vi "00 Main (three phase) (2017).vi"() -> ()   [LabVIEW 2017]
uses:
  <vilib>/DAQmx/read.llb/DAQmx Read (Analog 1D Wfm NChan NSamp).vi
  <vilib>/DAQmx/miscellaneous.llb/DAQmx Fill In Error Info.vi
panel:
  out "Error out (DAQ Loop)":errorcluster
  out "DAQ Loop Iterations":i32
  out "Raw DAQ Output":dynamicdata(graph)=[{"t0"=timestamp(3367839419.335167 s since 1904-01-01), "dt"=0.00016666666666666663, "Y"=array[240 elements], "attributes"=variant("NI_ChannelName"=variant(string "Voltage_0"), "NI_UnitDescription"=variant(string "Volts"))}, {"t0"=timestamp(3367839419.3351874 s since 1904-01-01), "dt"=0.00016666666666666663, "Y"=array[240 elements], "attributes"=variant("NI_ChannelName"=variant(string "Voltage_1"), "NI_UnitDescription"=variant(string "Volts"))}, {"t0"=timestamp(3367839419.3352084 s since 1904-01-01), "dt"=0.00016666666666666663, "Y"=array[240 elements], "attributes"=variant("NI_ChannelName"=variant(string "Voltage_2"), "NI_UnitDescription"=variant(string "Volts"))}]
  in  "All Stop!":bool
  out "Frequency 2":dynamicdata(graph)=[{"t0"=timestamp(3424329819.6880417 s since 1904-01-01), "dt"=0.00016666666666666663, "Y"=[50.00644377121546], "attributes"=variant("NI_ChannelName"=variant(string "Detected Frequency"))}, {"t0"=timestamp(3424329819.6880627 s since 1904-01-01), "dt"=0.00016666666666666663, "Y"=[49.993846178541475], "attributes"=variant("NI_ChannelName"=variant(string "Detected Frequency"))}, {"t0"=timestamp(3424329819.6880836 s since 1904-01-01), "dt"=0.00016666666666666663, "Y"=[49.994041382621866], "attributes"=variant("NI_ChannelName"=variant(string "Detected Frequency"))}] caption="Frequency"
  out "Phase 2":dynamicdata(graph)=[{"t0"=timestamp(3424329819.6880417 s since 1904-01-01), "dt"=0.00016666666666666663, "Y"=[-19.090260250465658], "attributes"=variant("NI_ChannelName"=variant(string "Detected Phase"))}, {"t0"=timestamp(3424329819.6880627 s since 1904-01-01), "dt"=0.00016666666666666663, "Y"=[-138.45601955575555], "attributes"=variant("NI_ChannelName"=variant(string "Detected Phase"))}, {"t0"=timestamp(3424329819.6880836 s since 1904-01-01), "dt"=0.00016666666666666663, "Y"=[102.37498697247455], "attributes"=variant("NI_ChannelName"=variant(string "Detected Phase"))}] caption="Frequency"
  out "Frequency":dbl format="%.2f"
  out "Amplitude":dbl format="%.2f"
  out "Phase":dbl format="%.2f"
  out "Acquisition Time":timestamp
  out "Voltage Waveform":dynamicdata(graph)=[{"t0"=timestamp(3424329819.638042 s since 1904-01-01), "dt"=0.00016666666666666663, "Y"=array[300 elements]}, {"t0"=timestamp(3424329819.6380625 s since 1904-01-01), "dt"=0.00016666666666666663, "Y"=array[300 elements]}, {"t0"=timestamp(3424329819.6380835 s since 1904-01-01), "dt"=0.00016666666666666663, "Y"=array[300 elements]}]
  out "IP":string
  out "Port":i32
  out "Transmitted Data":string
  out "Stop":bool
  out "Elements in Acquisition Buffer":i32
  # "V1.2 - PFI0 (Three Phase)"
  # "50.5"
  # "49.5"
  # "The code and design of this VI are licensed \nunder the terms of the New BSD License.\nPlease see the VI documentation or License.txt\nfor more details.\n\nCopyright (c) 2012, David Laverty\nwww.OpenPMU.org"
  # "180"
  # "-180"
  # "Configuration Information:\n\nThe ID and IP address to which the OpenPMU sends data is configured by 'C:\\PMUconfig.ini'.  If this doesn't exist, create it.\n\nCopy and paste the blue text below without the dashed lines into PMUconfig.ini.\n\n[Telecoms]\nID=PMU123\nIP=192.168.1.100\nPort=40001\n\nIP and Port may be any values within normal IPv4 range.  ID should be six alpha-numeric characters."
  # "Debug Stuff ( you're not supposed to find this :P )"
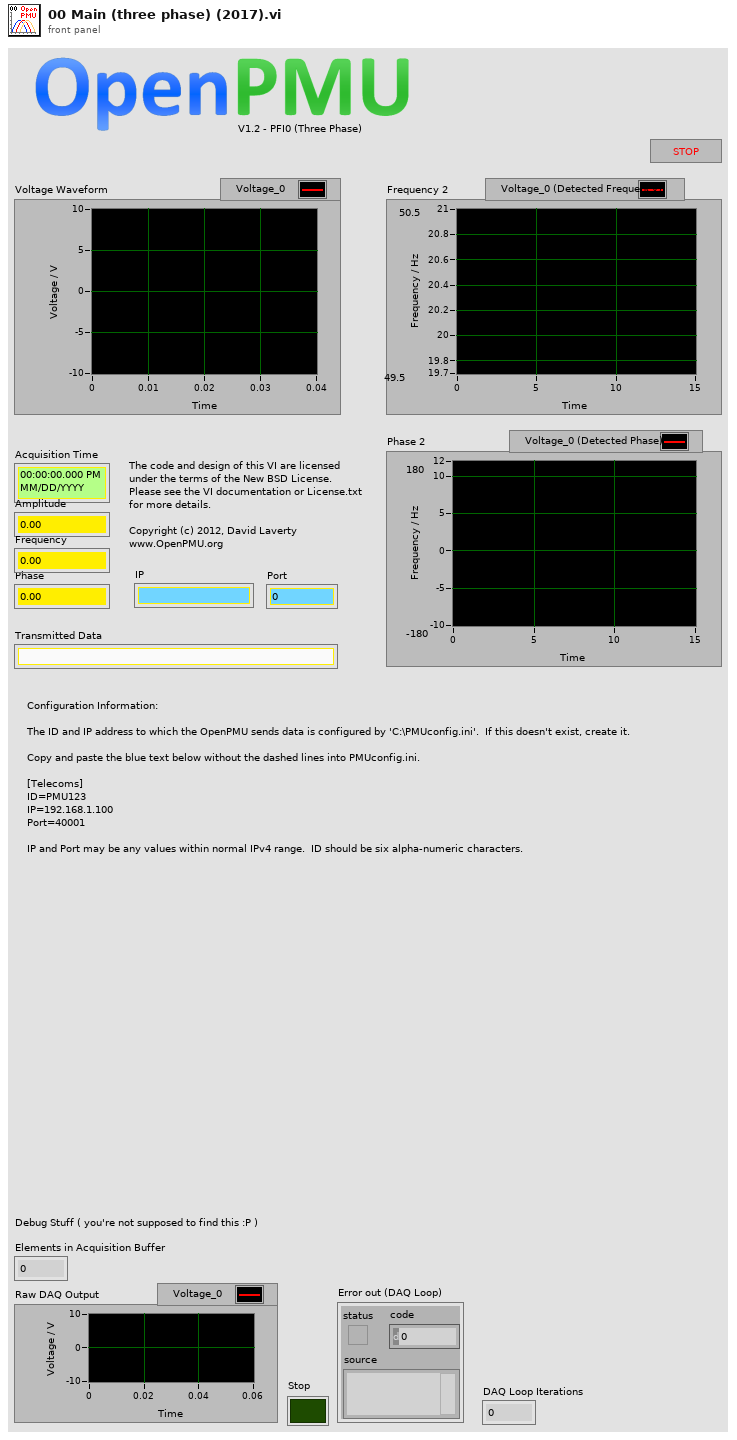
[diagram p1: front panel]
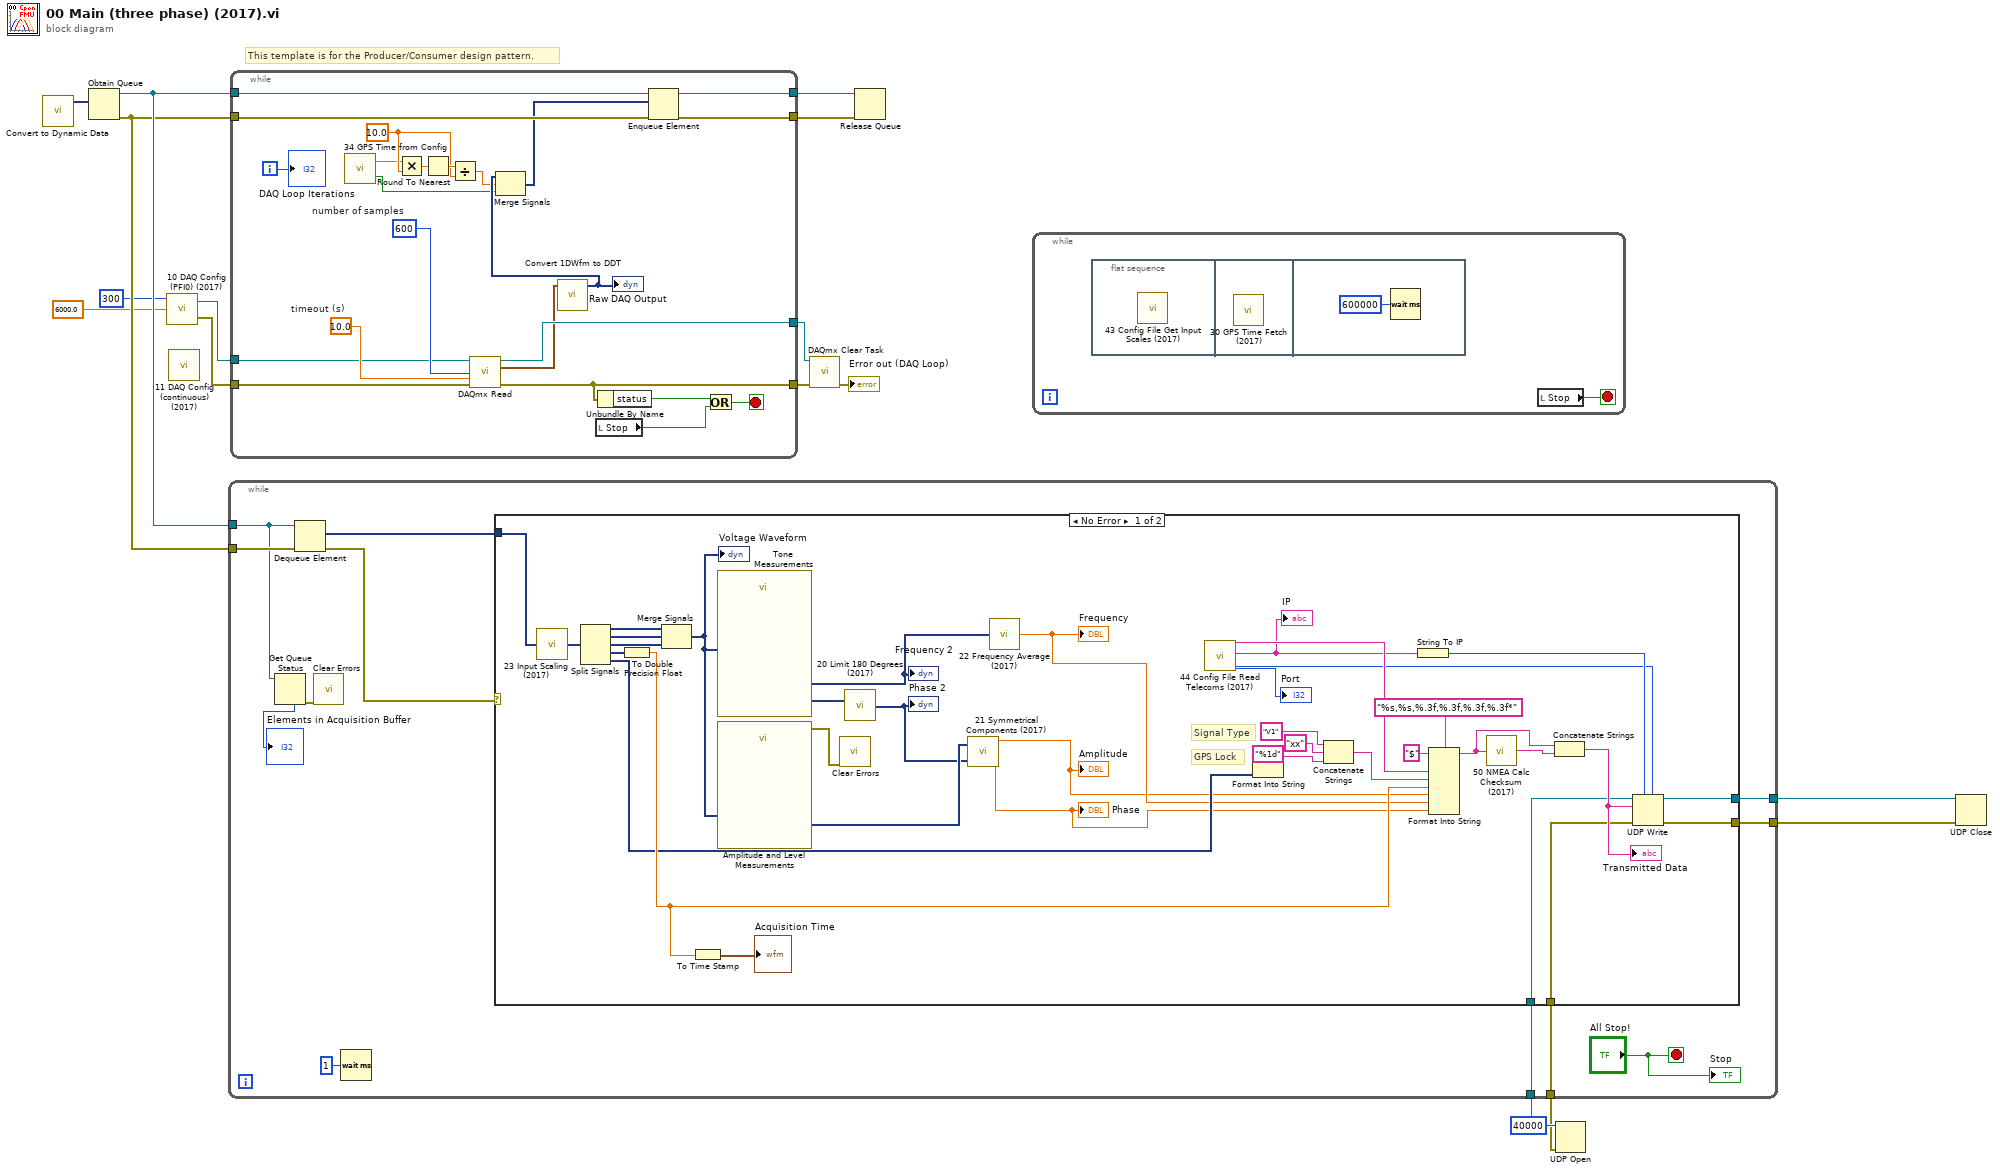
[diagram p0: block diagram]
diagram:
  # "This template is for the Producer/Consumer design pattern."
  n1 = call "Convert to Dynamic Data"() -> ("Dynamic Data Type"=w14:dynamicdata)  [unwired: 4 in]
  n2 = Obtain Queue(element data type=w14) -> (queue out=w11:refnum<queue>, error out=w10:errorcluster)  [unwired: 4 in, 1 out]
  n3 = call "10 DAQ Config (PFI0) (2017).vi"("rate"=6000.0, "number of samples"=300) -> ("Error Out"=w1:errorcluster, "task out"=w2:refnum<k21>)  [unwired: 1 in]
  n4 = call "11 DAQ Config (continuous) (2017).vi"() -> ()  [unwired: 1 in, 2 out]
  n5 = while {
    tunnel: w1 -> [w26]
    tunnel: w2 -> [w27]
    tunnel: [w37] -> w17
    tunnel: [w36] -> w16
    tunnel: w11 -> [w31]
    tunnel: w10 -> [w30]
    tunnel: [w29] -> w13
    tunnel: [w28] -> w12
    i -> [w35]
    stop <- w34 stop-if-true
    w20 = 10.0 ("y")
    w38 = 10.0  # timeout (s)
    w40 = 600  # number of samples
    n6 = call "34 GPS Time from Config.vi"() -> ("GPS Lock"=w18:bool, "Time"=w19:dbl)  [unwired: 2 in]
    n7 = Multiply(x=w19, y=w20) -> (x*y=w23:dbl)
    n8 = Round To Nearest(number=w23) -> (nearest integer value=w22:dbl)
    n9 = Divide(x=w22, y=w20) -> (x/y=w21:dbl)
    n10 = call-poly <vilib>:"DAQmx Read.vi"("task/channels in"=w27, "number of samples per channel"=w40, "timeout"=w38, "error in"=w26) -> ("task out"=w37:refnum<k21>, "data"=w33:waveform(dbl)[], "error out"=w36:errorcluster)  [unwired: 9 in]
    n11 = call <vilib>:"Convert 1DWfm to DDT.vi"("Array of Waveforms"=w33) -> ("Dynamic Data Type"=w25:dynamicdata)  [unwired: 3 in]
    "Raw DAQ Output" <- w25
    n12 = Merge Signals(w25, w21, w18) -> (w24:dynamicdata)
    n13 = local read "Stop"() -> (w32:bool)
    n14 = Unbundle By Name(w36) -> ("status"=w39:bool)
    n15 = Enqueue Element(queue=w31, element=w24, error in (no error)=w30) -> (queue out=w29:refnum<queue>, error out=w28:errorcluster)  [unwired: 1 in, 1 out]
    n16 = Or(x=w39, y=w32) -> (x .or. y?=w34:bool)
    "DAQ Loop Iterations" <- w35
  }
  n17 = call <vilib>:"DAQmx Clear Task.vi"("task in"=w17, "error in"=w16) -> ("error out"=→"Error out (DAQ Loop)":errorcluster)  [unwired: 13 in]
  n18 = Release Queue(queue=w13, error in (no error)=w12) -> ()  [unwired: 1 in, 3 out]
  n19 = while {
    stop <- w41 stop-if-true
    n20 = flat-sequence {
      frame #0 {
        n21 = call "43 Config File Get Input Scales (2017).vi"() -> ()  [unwired: 1 in]
      }
      frame #1 {
        n22 = call "30 GPS Time Fetch (2017).vi"() -> ()  [unwired: 1 in]
      }
      frame #2 {
        n23 = Wait (ms)(milliseconds to wait=u32 600000) -> ()  [unwired: 1 out]
      }
    }
    n24 = local read "Stop"() -> (w41:bool)
  }
  n25 = UDP Open(11:u16 40000 ("port")) -> (port=w8:refnum<k16>, 0:w7:errorcluster)  [unwired: 4 in, 1 out]
  n26 = while {
    tunnel: w11 -> [w48]
    tunnel: w10 -> [w50]
    tunnel: w8 -> [w47]
    tunnel: w7 -> [w46]
    tunnel: [w45] -> w6
    tunnel: [w44] -> w5
    stop <- "All Stop!" stop-if-true
    n27 = Get Queue Status(queue=w48) -> (error out=w43:errorcluster, # elements in queue=→"Elements in Acquisition Buffer":i32)  [unwired: 2 in, 6 out]
    n28 = Dequeue Element(queue=w48, error in (no error)=w50) -> (element=w51:dynamicdata, error out=w52:errorcluster)  [unwired: 1 in, 2 out]
    n29 = call <vilib>:"Clear Errors.vi"("error in (no error)"=w43) -> ()  [unwired: 5 in, 2 out]
    n30 = Wait (ms)(milliseconds to wait=u32 1) -> ()  [unwired: 1 out]
    n31 = case shown="No Error" w52 {
      tunnel: w51 -> [w56 _]
      tunnel: w47 -> [w84 w92]
      tunnel: w46 -> [w83 w91]
      tunnel: [w82 w92] -> w45
      tunnel: [w81 w91] -> w44
      frame No Error {
        # "GPS Lock"
        # "Signal Type"
        n32 = call "23 Input Scaling (2017).vi"("Input (Raw)"=w56) -> ("Output (Scaled)"=w55:dynamicdata)
        n33 = Split Signals(w55) -> (w69:dynamicdata, w70:dynamicdata, w71:dynamicdata, w80:dynamicdata, w78:dynamicdata)  [unwired: 5 in]
        n34 = To Double Precision Float(number=w80) -> (double precision float=w79:dbl)
        n35 = Merge Signals(w69, w70, w71) -> (w72:dynamicdata)
        "Voltage Waveform" <- w72
        n36 = To Time Stamp(1:w79) -> (0:→"Acquisition Time":timestamp)
        n37 = call "Tone Measurements"("Signals"=w72) -> ("Phase"=w68:dynamicdata, "Frequency"=w67:dynamicdata)  [unwired: 7 in, 2 out]
        "Frequency 2" <- w67
        n38 = call "Amplitude and Level Measurements"("Signals"=w72) -> ("Cycle RMS"=w65:dynamicdata, "error out"=w90:errorcluster)  [unwired: 13 in]
        n39 = call <vilib>:"Clear Errors.vi"("error in (no error)"=w90) -> ()  [unwired: 5 in, 2 out]
        n40 = call "20 Limit 180 Degrees (2017).vi"("Angle In"=w68) -> ("Angle Out"=w64:dynamicdata)
        "Phase 2" <- w64
        n41 = call "21 Symmetrical Components (2017).vi"("Amplitude"=w65, "Phase"=w64) -> ("V1"=w63:dbl, "Theta1"=w62:dbl)  [unwired: 4 out]
        "Amplitude" <- w63
        "Phase" <- w62
        n42 = call "22 Frequency Average (2017).vi"("Frequency"=w67) -> ("Numeric"=w66:dbl)
        "Frequency" <- w66
        n43 = call "44 Config File Read Telecoms (2017).vi"() -> ("Port"=w57:i32, "IP"=w58:string, "ID"=w59:string)  [unwired: 3 in]
        "IP" <- w58
        "Port" <- w57
        n44 = Format Into String(format string="%1d", w78) -> (resulting string=w73:string)  [unwired: 2 in, 1 out]
        n45 = Concatenate Strings("V1" ("input 2"), "xx" ("string"), w73) -> (w75:string)
        n46 = String To IP(1:w58) -> (0:w86:u32)
        n47 = Format Into String(format string="%s,%s,%.3f,%.3f,%.3f,%.3f*", initial string="$", w59, w75, w79, w63, w66, w62) -> (resulting string=w61:string)  [unwired: 1 in, 1 out]
        n48 = call "50 NMEA Calc Checksum (2017).vi"("GPS String"=w61) -> ("hex integer string"=w60:string)  [unwired: 1 in, 1 out]
        n49 = Concatenate Strings(w61, w60) -> (w85:string)
        "Transmitted Data" <- w85
        n50 = UDP Write(address=w86, port or service name=w57, connection ID=w84, data in=w85, 8:w83) -> (error out=w81:errorcluster, 3:w82:refnum<k16>)  [unwired: 1 in]
      }
      frame Error {
      }
    }
    "Stop" <- "All Stop!"
  }
  n51 = UDP Close(connection ID=w6, 8:w5) -> ()  [unwired: 2 out]
